vi "Header Footer Transform Header Footer [ ] V2.vi"(7 "Header or Footer [ ]":T15, 11 "error in (no error)":errorcluster) -> (8 "Header or Footer Complete Cluster":T1, 15 "error out":errorcluster)   [LabVIEW 2019]
doc: "Version 1.0\nDeveloped by Jean-Marc Simard\nCopyright © 2010, Exaprom Inc.\nAll rights reserved.\nLicense: BSD\n\nWith iTextSharp 4.1.6 (http://itextsharp.sourceforge.net)\nunder Mozilla Public License Version 1.1\n(http://www.mozilla.org/MPL/MPL-1.1.html)"
uses:
  C:/Program Files/National Instruments/LabVIEW 2019/user.lib/Exaprom PDF/DLL/itextsharp.dll
  DLL/itextsharp.dll
  <userlib>/Exaprom PDF/Controls/Header, Footer and Watermark Controls/Header Footer Type.ctl
  <userlib>/Exaprom PDF/Controls/Header, Footer and Watermark Controls/Header footer horiz alignment.ctl
  <userlib>/Exaprom PDF/Controls/Table Controls/Cell Vertical alignment.ctl
  <userlib>/Exaprom PDF/Controls/Header, Footer and Watermark Controls/Page number.ctl
  <userlib>/Exaprom PDF/Controls/Font Controls/Font size.ctl
  <userlib>/Exaprom PDF/Controls/Font Controls/Font color.ctl
  <userlib>/Exaprom PDF/Controls/Header, Footer and Watermark Controls/Header Footer Line.ctl
  <userlib>/Exaprom PDF/Controls/Header, Footer and Watermark Controls/Header Footer Cluster with references.ctl
  <userlib>/Exaprom PDF/Controls/Header, Footer and Watermark Controls/Header or Footer Position.ctl
  <userlib>/Exaprom PDF/Controls/Text Controls/Line spacing.ctl
  <userlib>/Exaprom PDF/Controls/Text Controls/Unicode/Type and run direction.ctl
  <userlib>/Exaprom PDF/Controls/Font Controls/Type and encoding.ctl
  <userlib>/Exaprom PDF/Controls/Font Controls/Font complete cluster horizontal.ctl
  <userlib>/Exaprom PDF/Controls/Header, Footer and Watermark Controls/Header Footer Complete Cluster.ctl
  <userlib>/Exaprom PDF/Controls/Header, Footer and Watermark Controls/Header or Footer.ctl
  <userlib>/Exaprom PDF/LV Class/Header and Footer Class/VIs/Controls/Header Footer cluster V2.ctl
  <userlib>/Exaprom PDF/LV Class/Header and Footer Class/VIs/Controls/Header Footer [ ] V2.ctl
panel:
  # "X"
  # "Y"
  # "X"
  # "Y"
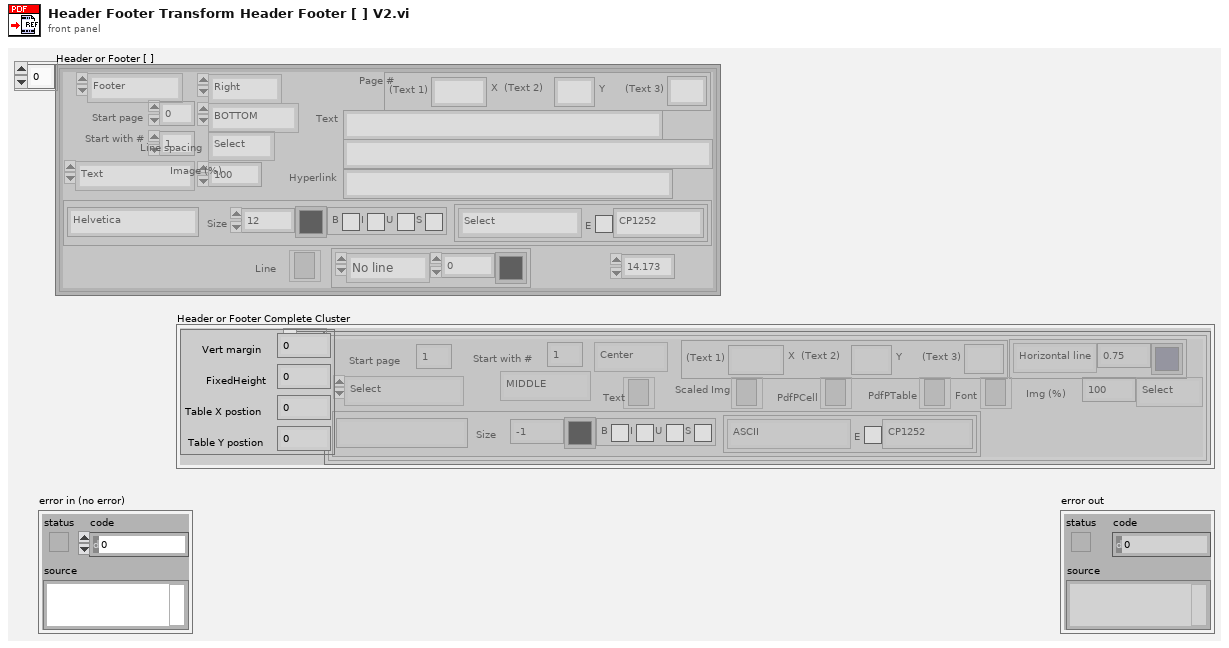
[diagram p1: front panel]
types:
  T1 = typedef "Header Footer Complete Cluster.ctl" = cluster{"Table position":T2, "Header Footer Cluster with references [ ]":T3[]}
  T2 = typedef "Header or Footer Position.ctl" = cluster{"Vert margin":dbl, "FixedHeight":dbl, "Table X postion":dbl, "Table Y postion":dbl}
  T3 = typedef "Header Footer Cluster with references.ctl" = cluster{"Start page":i32, "Type":T4, "Start with #":i32, "Alignment":T5, "Vertical Alignement":T6, "Page #":T7, "Text":refnum<k24>, "Scaled Img":refnum<k24>, "PdfPCell":refnum<k24>, "PdfPTable":refnum<k24>, "Font Cluster":T8, "Font ":refnum<k24>, "Img (%)":sgl, "Line":cluster{"Line":T13, "Thickness (points)":sgl, "Colour":T10}, "Line spacing":T14}
  T4 = typedef "Header Footer Type.ctl" = enum16{"Select", "Text", "Text + hyperlink", "Page number", "Image", "Image + hyperlink"}
  T5 = typedef "Header footer horiz alignment.ctl" = enum16{"Left", "Center", "Right"}
  T6 = typedef "Cell Vertical alignment.ctl" = enum16{"TOP", "MIDDLE", "BOTTOM"}
  T7 = typedef "Page number.ctl" = cluster{"Text 1":string, "Text 2":string, "Text 3":string}
  T8 = typedef "Font complete cluster horizontal.ctl" = cluster{"Name":string, "Size":T9, "Color":T10, "Style":cluster{"Bold":bool, "Italic":bool, "Underline":bool, "Strikeout":bool}, "Type":T11}
  T9 = typedef "Font size.ctl" = sgl
  T10 = typedef "Font color.ctl" = u32
  T11 = typedef "Type and encoding.ctl" = cluster{"Type&direction":T12, "Embedded":bool, "Encoding":string}
  T12 = typedef "Type and run direction.ctl" = enum16{"Select", "ASCII", "UTF-16", "UTF-16 (default)", "UTF-16 (LTR)", "UTF-16 (RTL)"}
  T13 = typedef "Header Footer Line.ctl" = enum16{"No line", "Horizontal line"}
  T14 = typedef "Line spacing.ctl" = enum16{"Select", "1.0", "1.5", "2.0"}
  T15 = typedef "Header Footer [ ] V2.ctl" = T16[]
  T16 = typedef "Header Footer cluster V2.ctl" = cluster{"Header or Footer":T17, "Start page":i32, "Start with #":i32, "Type":T4, "Alignment":T5, "Vertical Alignement":T6, "Line spacing":T14, "Image (%)":sgl, "Page #":T7, "Text":string, "Path":string, "Font":T8, "Font refnum":refnum<k24>, "Line":cluster{"Line":T13, "Thickness (points)":sgl, "Colour":T10}, "Vert margin":dbl, "Hyperlink":string}
  T17 = typedef "Header or Footer.ctl" = enum16{"Header", "Footer"}
  T18 = cluster{"Line":T13, "Thickness (points)":sgl, "Colour":T10}
  T19 = cluster{"Table position":T2, "Header Footer Cluster with references [ ]":T3[]}
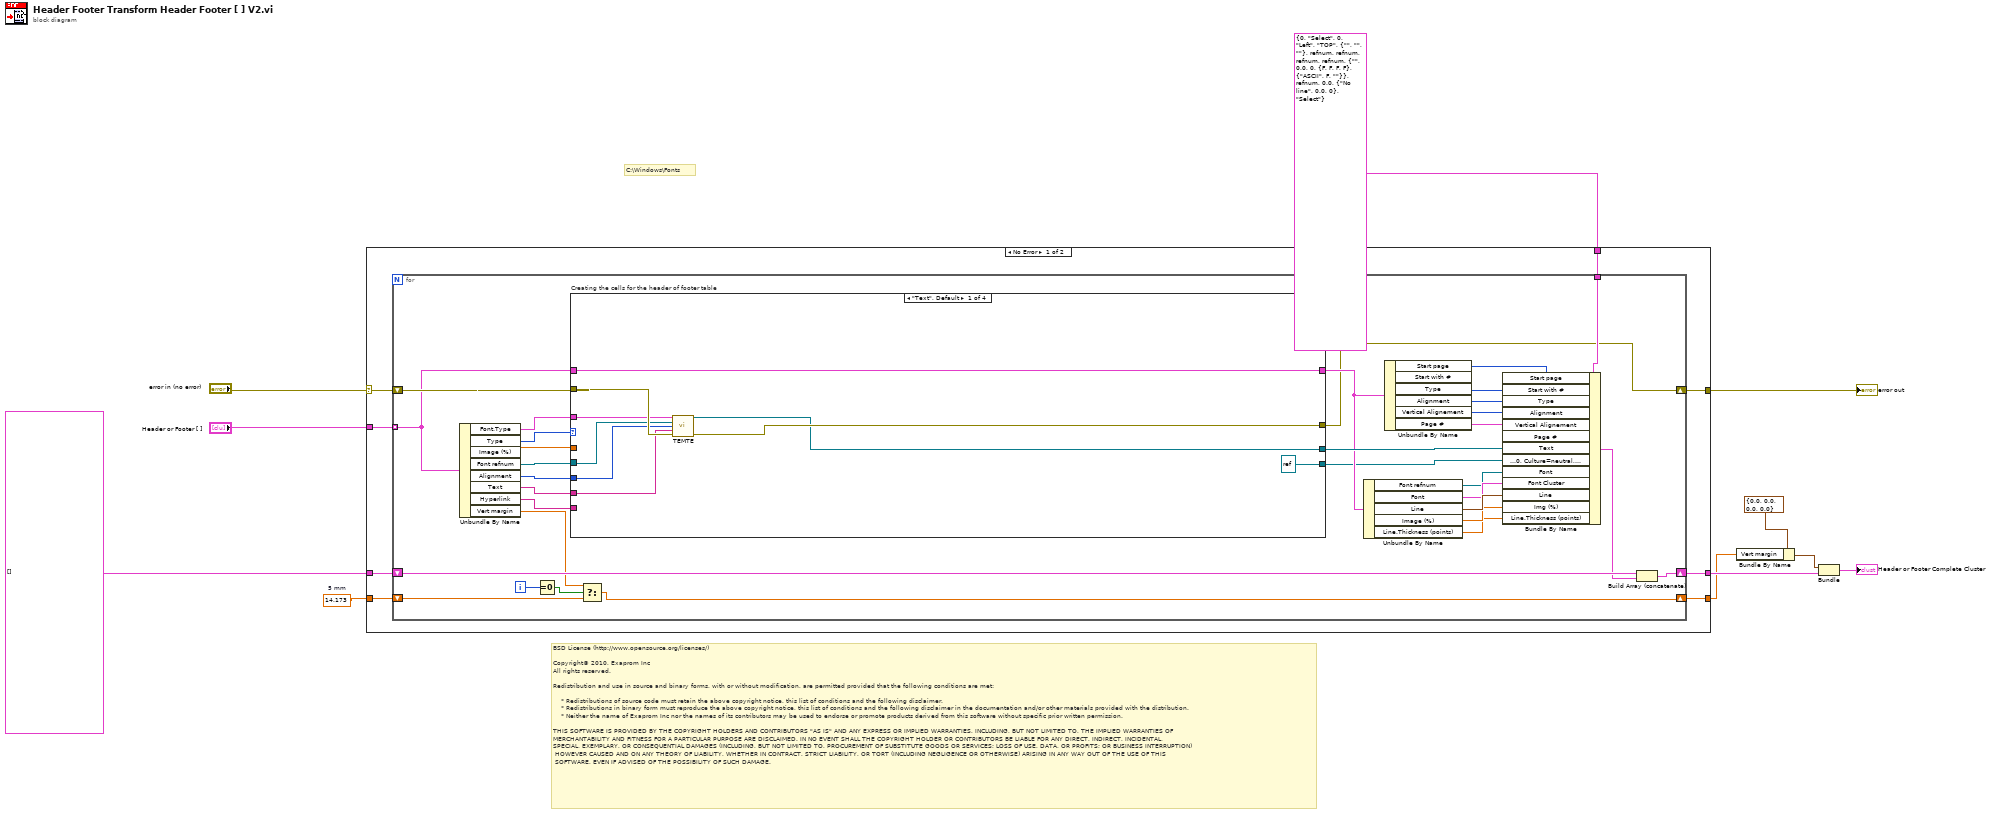
[diagram p0: block diagram]
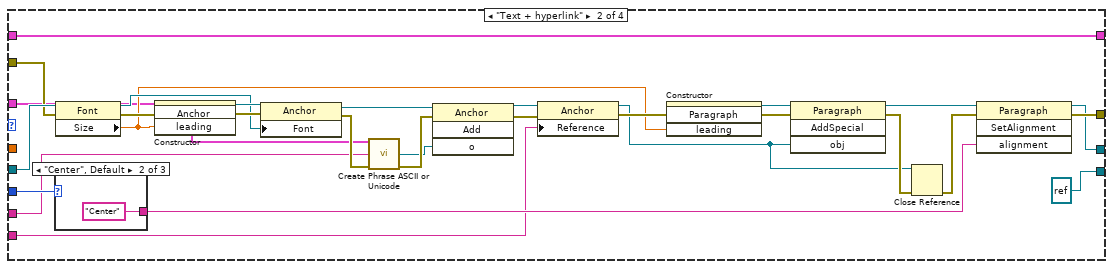
[diagram p2: hidden frame]
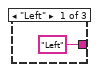
[diagram p3: hidden frame]
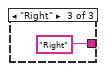
[diagram p4: hidden frame]
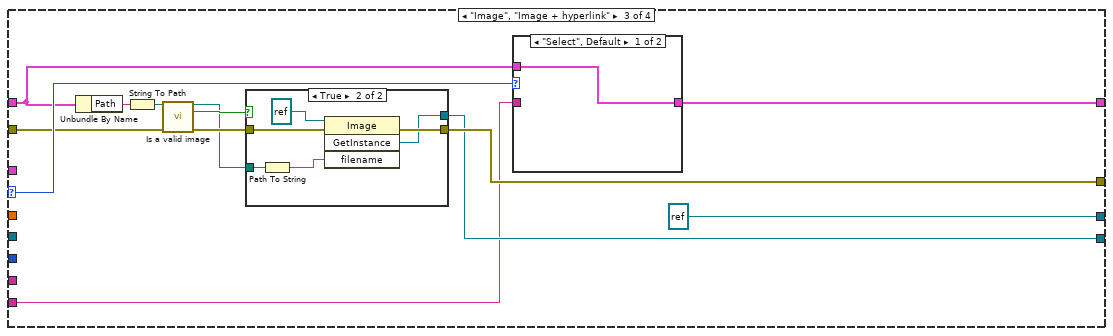
[diagram p5: hidden frame]
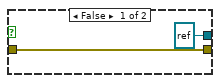
[diagram p6: hidden frame]
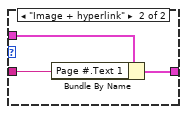
[diagram p7: hidden frame]
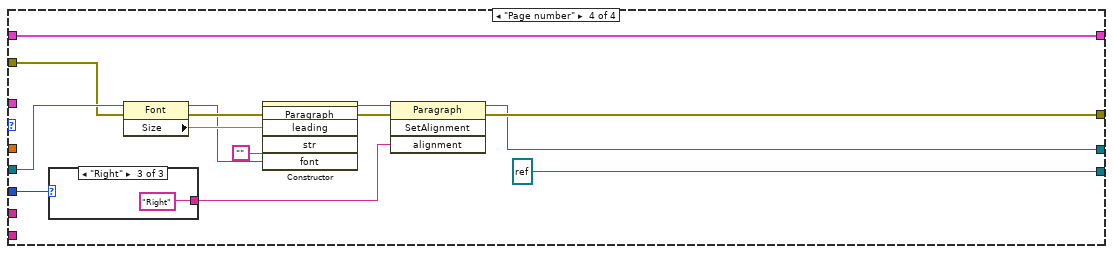
[diagram p8: hidden frame]
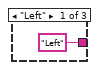
[diagram p9: hidden frame]
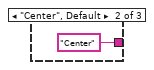
[diagram p10: hidden frame]
diagram:
  w4 = 14.173  # 5 mm
  # "C:\\Windows\\Fonts"
  # "BSD License (http://www.opensource.org/licenses/)\n\nCopyright© 2010, Exaprom Inc\nAll rights reserved.\n\nRedistribution and use in source and binary forms, with or without modification, are permitted provided that the following conditions are met:\n\n    * Redistributions of source code must retain the above copyright notice, this list of conditions and the following disclaimer.\n    * Redistributions in binary form must reproduce the above copyright notice, this list of conditions and the following disclaimer in the documentation and/or other materials provided with the distribution.\n    * Neither the name of Exaprom Inc nor the names of its contributors may be used to endorse or promote products derived from this software without specific prior written permission.\n\nTHIS SOFTWARE IS PROVIDED BY THE COPYRIGHT HOLDERS AND CONTRIBUTORS \"AS IS\" AND ANY EXPRESS OR IMPLIED WARRANTIES, INCLUDING, BUT NOT LIMITED TO, THE IMPLIED WARRANTIES OF \nMERCHANTABILITY AND FITNESS FOR A PARTICULAR PURPOSE ARE DISCLAIMED. IN NO EVENT SHALL THE COPYRIGHT HOLDER OR CONTRIBUTORS BE LIABLE FOR ANY DIRECT, INDIRECT, INCIDENTAL,\nSPECIAL, EXEMPLARY, OR CONSEQUENTIAL DAMAGES (INCLUDING, BUT NOT LIMITED TO, PROCUREMENT OF SUBSTITUTE GOODS OR SERVICES; LOSS OF USE, DATA, OR PROFITS; OR BUSINESS INTERRUPTION)\n HOWEVER CAUSED AND ON ANY THEORY OF LIABILITY, WHETHER IN CONTRACT, STRICT LIABILITY, OR TORT (INCLUDING NEGLIGENCE OR OTHERWISE) ARISING IN ANY WAY OUT OF THE USE OF THIS\n SOFTWARE, EVEN IF ADVISED OF THE POSSIBILITY OF SUCH DAMAGE."
  n1 = case shown="No Error" "error in (no error)" {
    selector: "error in (no error)" -> [w15 w138]
    tunnel: "Header or Footer [ ]" -> [w14 _]
    tunnel: [w19 w138] -> w11
    tunnel: T3 {"Start page"=0, "Type"=enum."Select", "Start with #"=0, "Alignment"=enum."Left", "Vertical Alignement"=enum."TOP", "Page #"={"Text 1"="", "Text 2"="", "Text 3"=""}, "Text"=refnum, "Scaled Img"=refnum, "PdfPCell"=refnum, "PdfPTable"=refnum, "Font Cluster"={"Name"="", "Size"=0.0, "Color"=0, "Style"={"Bold"=FALSE, "Italic"=FALSE, "Underline"=FALSE, "Strikeout"=FALSE}, "Type"={"Type&direction"=enum."ASCII", "Embedded"=FALSE, "Encoding"=""}}, "Font "=refnum, "Img (%)"=0.0, "Line"={"Line"=enum."No line", "Thickness (points)"=0.0, "Colour"=0}, "Line spacing"=enum."Select"} ("Header Footer Cluster with references") -> [w18 _]
    tunnel: T3[] [] ("Header Footer Cluster with references [ ]") -> [w17 w137]
    tunnel: [w16 w137] -> w6
    tunnel: [w13 w136] -> w1
    tunnel: w4 -> [w12 w136]
    frame No Error {
      n2 = for {
        tunnel: w14 -> [w38] mode=indexing
        tunnel: w18 -> [w47]
        shift-right: [w40] -> w16
        shift-left: w17 -> [w39]
        shift-right: [w33] -> w19
        shift-left: w15 -> [w36]
        shift-right: [w25] -> w13
        shift-left: w12 -> [w26]
        i -> [w28]
        n3 = Unbundle By Name(w38) -> ("Font.Type"=w22:T11, "Type"=w49:T4, "Image (%)"=w50:sgl, "Font refnum"=w52:refnum<k24>, "Alignment"=w51:T5, "Text"=w48:string, "Hyperlink"=w20:string, "Vert margin"=w21:dbl)
        n4 = Equal To 0?(x=w28) -> (x = 0?=w27:bool)
        n5 = case "Creating the cells for the header of footer table" shown="\"Text\", Default" w49 {
          selector: w49 -> [_ _ w104 _]
          tunnel: w38 -> [w60 w85 w99 w127]
          tunnel: w52 -> [w57 w90 _ w132]
          tunnel: w51 -> [w56 w89 _ w131]
          tunnel: w50 -> [_ _ _ _]
          tunnel: w48 -> [w55 w63 _ _]
          tunnel: w36 -> [w59 w88 w96 w130]
          tunnel: [w53 w76 refnum<k24> refnum ("new reference") w126] -> w41
          tunnel: [refnum<k24> refnum ("GetInstanceImage OUT") refnum<k24> refnum ("GetInstanceImage OUT") w102 refnum<k24> refnum ("GetInstanceImage OUT")] -> w35
          tunnel: [w54 w86 w105 w129] -> w33
          tunnel: [w60 w85 w103 w127] -> w37
          tunnel: w22 -> [w58 w62 _ _]
          tunnel: w20 -> [_ w75 w94 _]
          frame "Text", Default {
            n6 = call <userlib>:"TEMTE.vi"("Type and run direction"=w58, "Font refnum"=w57, "Alignment"=w56, "Text"=w55, "error in (no error)"=w59) -> ("Paragraph"=w53:refnum<k24>, "error out"=w54:errorcluster)  [unwired: 9 in]
          }
          frame "Text + hyperlink" {
            n7 = case shown="\"Center\", Default" w89 {
              tunnel: ["Left" "Center" "Right"] -> w84
              frame "Left" {
              }
              frame "Center", Default {
              }
              frame "Right" {
              }
            }
            n8 = property class="Font"(reference=w90, error in=w88) -> (reference out=w70:refnum<k24>, error out=w71:errorcluster, "Size"=w69:sgl)
            n9 = constructor class="Anchor"(error in=w71, "leading"=w69) -> (reference out=w74:refnum<k24>, error out=w73:errorcluster)  [unwired: 2 in, 2 out]
            n10 = property class="Anchor"(reference=w74, error in=w73, "Font"=w70) -> (reference out=w72:refnum<k24>, error out=w66:errorcluster)
            n11 = call <userlib>:"Create Phrase ASCII or Unicode.vi"("Character type"=w62, "Text"=w63, "error in (no error)"=w66) -> ("Phrase refnum"=w64:refnum<k24>, "error out"=w65:errorcluster)  [unwired: 10 in, 1 out]
            n12 = invoke class="Anchor" method="Add"(reference=w72, error in=w65, "o"=w64) -> (reference out=w67:refnum<k24>, error out=w68:errorcluster)  [unwired: 1 in, 2 out]
            n13 = property class="Anchor"(reference=w67, error in=w68, "Reference"=w75) -> (reference out=w77:refnum<k24>, error out=w83:errorcluster)
            n14 = constructor class="Paragraph"(error in=w83, "leading"=w69) -> (reference out=w80:refnum<k24>, error out=w81:errorcluster)  [unwired: 2 in, 2 out]
            n15 = invoke class="Paragraph" method="AddSpecial"(reference=w80, error in=w81, "obj"=w77) -> (reference out=w82:refnum<k24>, error out=w79:errorcluster)  [unwired: 1 in, 2 out]
            n16 = Close Reference(reference=w77, error in (no error)=w79) -> (error out=w78:errorcluster)
            n17 = invoke class="Paragraph" method="SetAlignment"(reference=w82, error in=w78, "alignment"=w84) -> (reference out=w76:refnum<k24>, error out=w86:errorcluster)  [unwired: 1 in, 2 out]
          }
          frame "Image", "Image + hyperlink" {
            n18 = Unbundle By Name(w99) -> ("Path"=w100:string)
            n19 = String To Path(string=w100) -> (path=w101:path)
            n20 = call <userlib>:"Is a valid image.vi"("Image path"=w101, "error in (no error)"=w96) -> ("dup path"=w95:path, "Valid Image?"=w98:bool, "error out"=w97:errorcluster)  [unwired: 11 out]
            n21 = case shown="True" w98 {
              tunnel: w95 -> [_ w113]
              tunnel: [w108 w112] -> w105
              tunnel: [refnum<k24> refnum ("GetInstance") w111] -> w102
              tunnel: w97 -> [w108 w110]
              frame False {
              }
              frame True {
                n22 = Path To String(path=w113) -> (string=w109:string)
                n23 = invoke class="Image" method="GetInstance"(reference=refnum<k24> refnum ("image"), error in=w110, "filename"=w109) -> (error out=w112:errorcluster, "GetInstance"=w111:refnum<k24>)  [unwired: 1 in, 2 out]
              }
            }
            n24 = case shown="\"Select\", Default" w104 {
              tunnel: [w115 w117] -> w103
              tunnel: w99 -> [w115 w118]
              tunnel: w94 -> [_ w116]
              frame "Select", Default {
              }
              frame "Image + hyperlink" {
                n25 = Bundle By Name(cluster=w118, "Page #.Text 1"=w116) -> (w117:T16)
              }
            }
          }
          frame "Page number" {
            n26 = case shown="\"Right\"" w131 {
              tunnel: ["Left" "Center" "Right"] -> w123
              frame "Left" {
              }
              frame "Center", Default {
              }
              frame "Right" {
              }
            }
            n27 = property class="Font"(reference=w132, error in=w130) -> (reference out=w120:refnum<k24>, error out=w122:errorcluster, "Size"=w121:sgl)
            n28 = constructor class="Paragraph"(error in=w122, "leading"=w121, "str"="", "font"=w120) -> (reference out=w124:refnum<k24>, error out=w119:errorcluster)  [unwired: 2 in, 4 out]
            n29 = invoke class="Paragraph" method="SetAlignment"(reference=w124, error in=w119, "alignment"=w123) -> (reference out=w126:refnum<k24>, error out=w129:errorcluster)  [unwired: 1 in, 2 out]
          }
        }
        n30 = Select(t=w21, s=w27, f=w26) -> (s? t:f=w25:dbl)
        n31 = Unbundle By Name(w37) -> ("Font refnum"=w30:refnum<k24>, "Font"=w31:T8, "Line"=w32:T18, "Image (%)"=w29:sgl, "Line.Thickness (points)"=w23:sgl)
        n32 = Unbundle By Name(w37) -> ("Start page"=w24:i32, "Start with #"=w46:i32, "Type"=w45:T4, "Alignment"=w44:T5, "Vertical Alignement"=w43:T6, "Page #"=w42:T7)
        n33 = Bundle By Name(cluster=w47, "Start page"=w24, "Start with #"=w46, "Type"=w45, "Alignment"=w44, "Vertical Alignement"=w43, "Page #"=w42, "Text"=w41, "Scaled Img"=w35, "Font"=w30, "Font Cluster"=w31, "Line"=w32, "Img (%)"=w29, "Line.Thickness (points)"=w23) -> (w34:T3)
        n34 = Build Array (concatenate)(w39, w34) -> (w40:T3[])
      }
    }
    frame Error {
    }
  }
  "error out" <- w11
  n35 = Bundle By Name(cluster=T2 {"Vert margin"=0.0, "FixedHeight"=0.0, "Table X postion"=0.0, "Table Y postion"=0.0} ("Table position"), "Vert margin"=w1) -> (w2:T2)
  n36 = Bundle("Table position"=w2, "Header Footer Cluster with references [ ]"=w6) -> (→"Header or Footer Complete Cluster":T19)  [unwired: 1 out]
